vi "Write Calibration.vi"(8 "error in (no error)":errorcluster, 10 "Calibration":T1, 11 "RP Communicator in":refnum<class "RP Communicator.lvclass">) -> (0 "error out":errorcluster, 3 "RP Communicator out":refnum<class "RP Communicator.lvclass">)   [LabVIEW 2024, in "RP Communicator.lvclass"]
uses:
  RP Communicator.lvclass
  RP Calibration.ctl
  RP Calibration 4ch.ctl
  RP Channel Calibration.ctl
  RP Filter 4ch.ctl
  RP Channel Filter.ctl
  RP Calibration 2ch.ctl
  RP Command.ctl
  RP Communicator.lvclass/RP Communicator.ctl
  RP Write Command TCP.vi
panel:
  out "length":i32
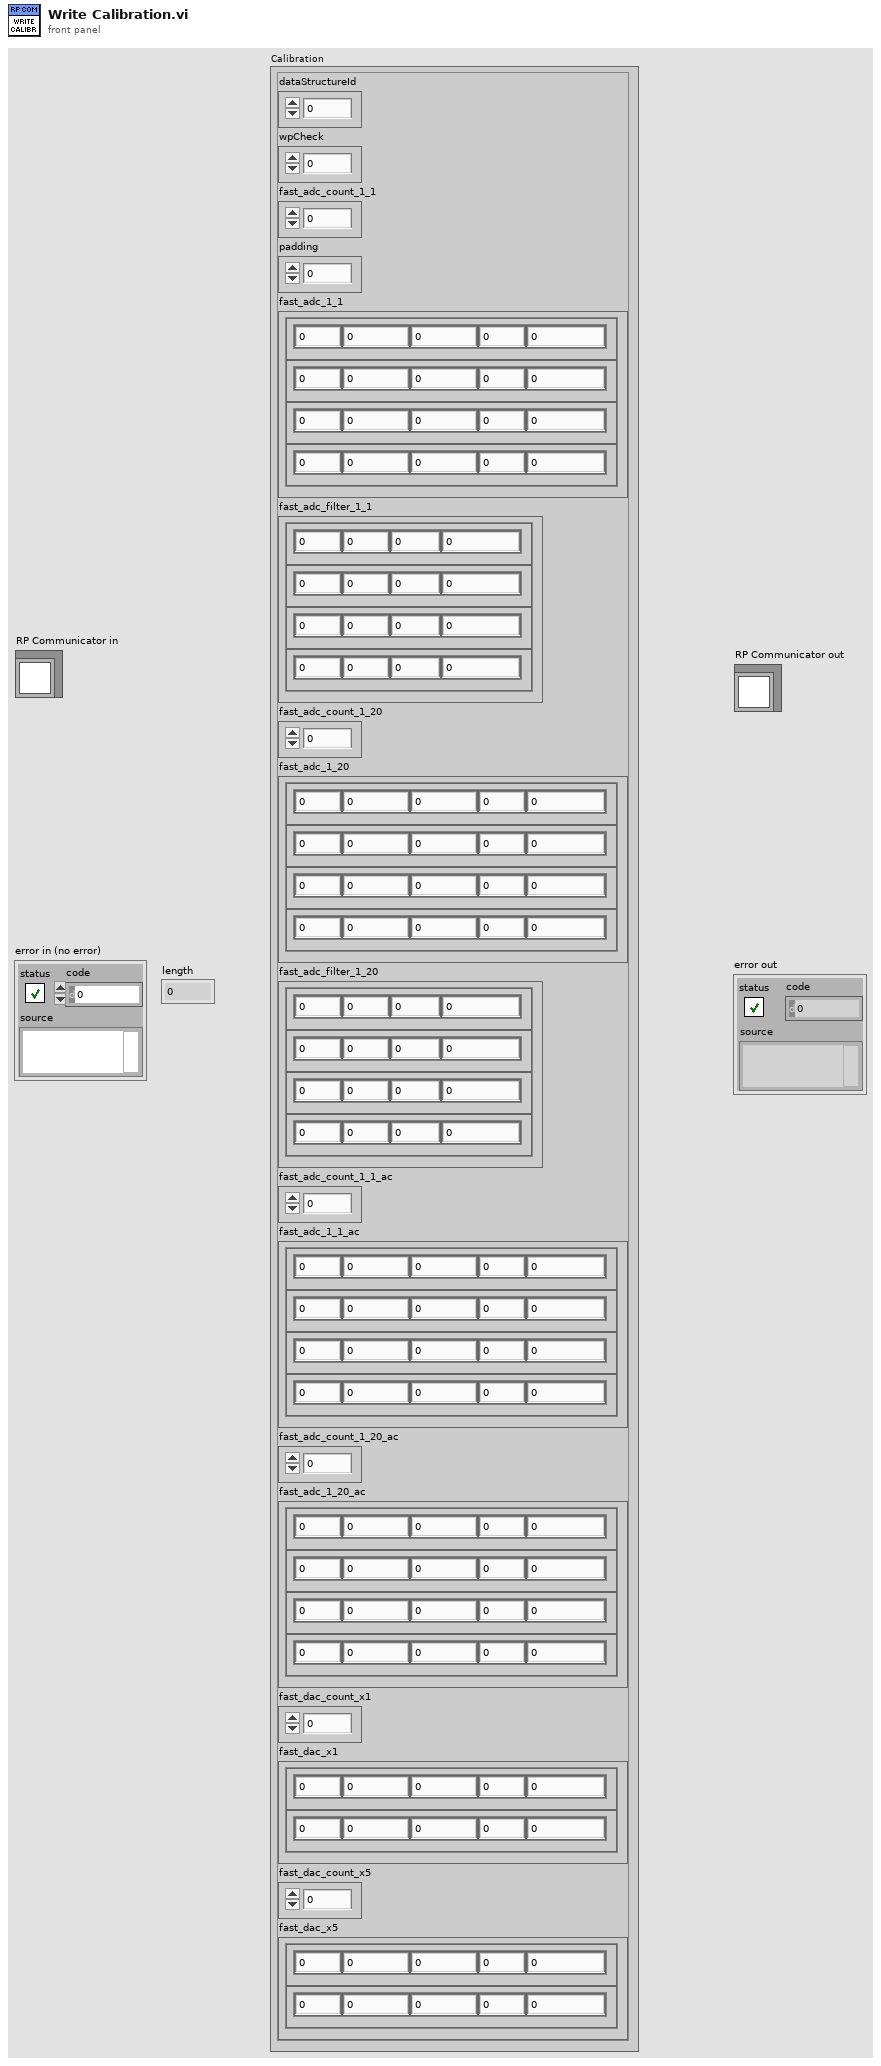
[diagram p1: front panel]
types:
  T1 = typedef "RP Calibration.ctl" = cluster{"dataStructureId":u8, "wpCheck":u8, "fast_adc_count_1_1":u16, "padding":u32, "fast_adc_1_1":T2, "fast_adc_filter_1_1":T4, "fast_adc_count_1_20":u64, "fast_adc_1_20":T2, "fast_adc_filter_1_20":T4, "fast_adc_count_1_1_ac":u64, "fast_adc_1_1_ac":T2, "fast_adc_count_1_20_ac":u64, "fast_adc_1_20_ac":T2, "fast_dac_count_x1":u64, "fast_dac_x1":T6, "fast_dac_count_x5":u64, "fast_dac_x5":T6}
  T2 = typedef "RP Calibration 4ch.ctl" = cluster{"ch_0":T3, "ch_1":T3, "ch_2":T3, "ch_3":T3}
  T3 = typedef "RP Channel Calibration.ctl" = cluster{"baseScale":sgl, "calibValue":u32, "offset":i32, "padding 2":i32, "gainCalc":dbl}
  T4 = typedef "RP Filter 4ch.ctl" = cluster{"ch_0":T5, "ch_1":T5, "ch_2":T5, "ch_3":T5}
  T5 = typedef "RP Channel Filter.ctl" = cluster{"aa":u32, "bb":u32, "pp":u32, "kk":u32}
  T6 = typedef "RP Calibration 2ch.ctl" = cluster{"ch_0":T3, "ch_1":T3}
  T7 = typedef "RP Command.ctl" = enum16{"Reset", "Read IDN", "Stop server", "Get status", "Get temperature", "Connect client", "Arm", "Software trigger", "Get whole buffer", "Get chunk", "System call", "Get config", "Set config", "Recieve data", "Recieve Calibartion", "Transmit data"}
  T8 = enum16{"big-endian, network order", "native, host order", "little-endian"}
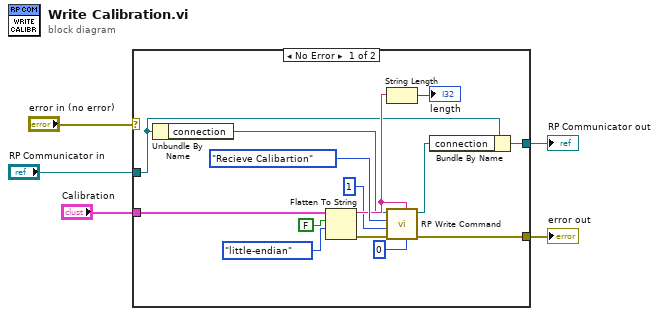
[diagram p0: block diagram]
diagram:
  n1 = case shown="No Error" "error in (no error)" {
    selector: "error in (no error)" -> [_ w21]
    tunnel: [w17 w21] -> w3
    tunnel: [w9 w20] -> w2
    tunnel: "RP Communicator in" -> [w8 w20]
    tunnel: "Calibration" -> [w14 _]
    frame No Error {
      n2 = Unbundle By Name(w8) -> ("connection"=w11:refnum<k5>)
      n3 = Flatten To String(anything=w14, prepend array or string size? (T)=FALSE, byte order (0:big-endian, network order)=T8."little-endian") -> (data string=w13:string, error out=w10:errorcluster)  [unwired: 1 in, 1 out]
      n4 = String Length(string=w13) -> (length=→"length":i32)
      n5 = call-poly "RP Write Command.vi"("bytes to read"=0, "Payload data"=w13, "Error In"=w10, "Command payload"=u64 1, "Command number"=RP_Command."Recieve Calibartion", "connection ID"=w11) -> ("Error Out"=w17:errorcluster, "connection ID out"=w7:refnum<k5>)  [unwired: 2 in, 2 out]
      n6 = Bundle By Name(cluster=w8, "connection"=w7) -> (w9:refnum<class "RP Communicator.lvclass">)
    }
    frame Error {
    }
  }
  "error out" <- w3
  "RP Communicator out" <- w2
